vi "final16.vi"() -> ()   [LabVIEW 2019]
uses:
  <vilib>/Instr/_visa.llb/VISA Configure Serial Port (Instr).vi
  <vilib>/Analysis/NI_AALBase.lvlib
  <vilib>/Analysis/NI_AALPro.lvlib
panel:
  out "Noise":dbl
  out "Relative errors array":dbl[](array[numeric])
  out "Absolute errors array":dbl[](array[numeric])
  out "Calibration - read data":dbl[][](array[numeric])
  out "Received data":string[][](array[string])
  out "slope_gain0":dbl
  out "intercept_gain0":dbl
  out "residue_gain0":dbl
  out "slope_gain2":dbl
  out "intercept_gain2":dbl
  out "residue_gain2":dbl
  out "slope_gain1":dbl
  out "intercept_gain1":dbl
  out "residue_gain1":dbl
  out "standard deviation":dbl format="%0.2f"
  out "variance":dbl format="%0.2f"
  out "mean":dbl format="%0.2f"
  out "Conversion [g]":dbl
  out "String passed to Arduino":string
  out "Received data array":dbl[](array[numeric])
  out "Debug array":string[](array[string])
  in  "Stop":bool
  in  "Cycles":dbl min=1.0 step=1.0
  in  "Start operation":bool
  in  "Function":u16(ring) items=["Read data ", "Compare different gains", "Execute calibration"]
  in  "Gain":u16(ring) items=["32", "64", "128"]
  in  "Arduino COM port":refnum<visa-resource-name>="COM6"
  # "Select all options, then press \"Start operation\" button"
  # "Nerd zone"
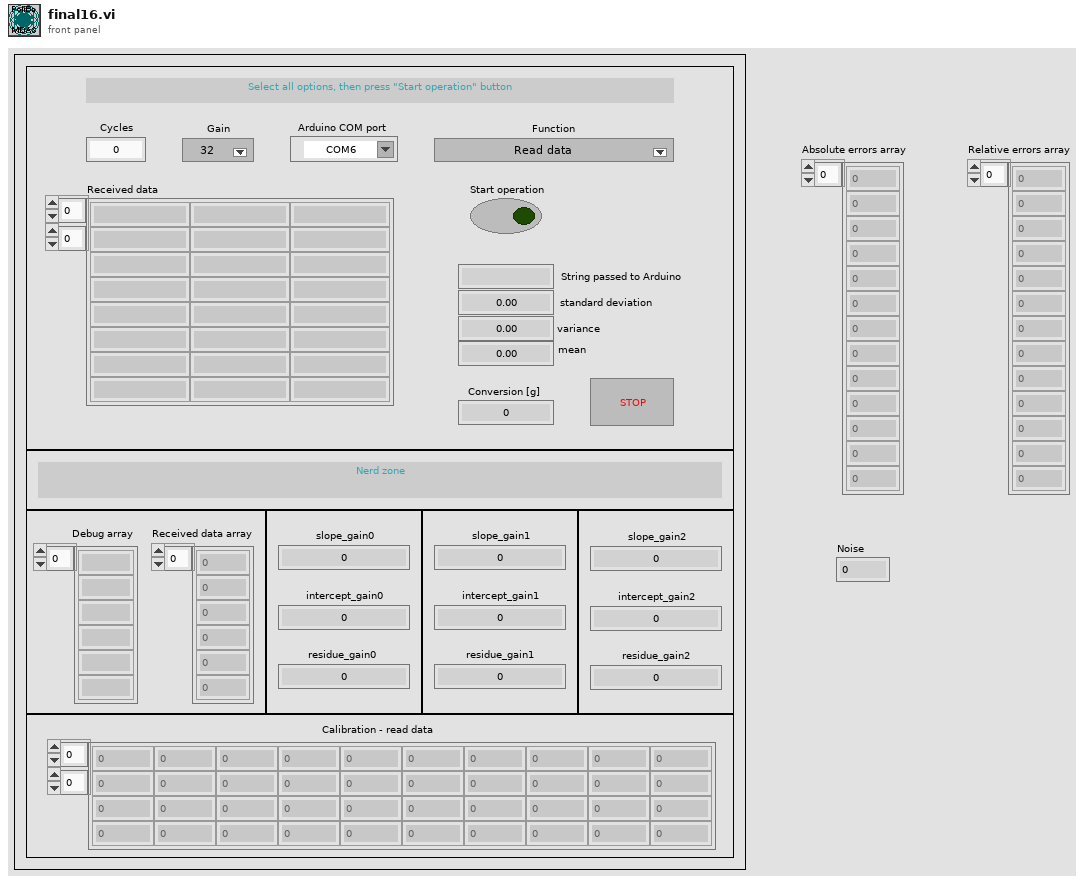
[diagram p1: front panel]
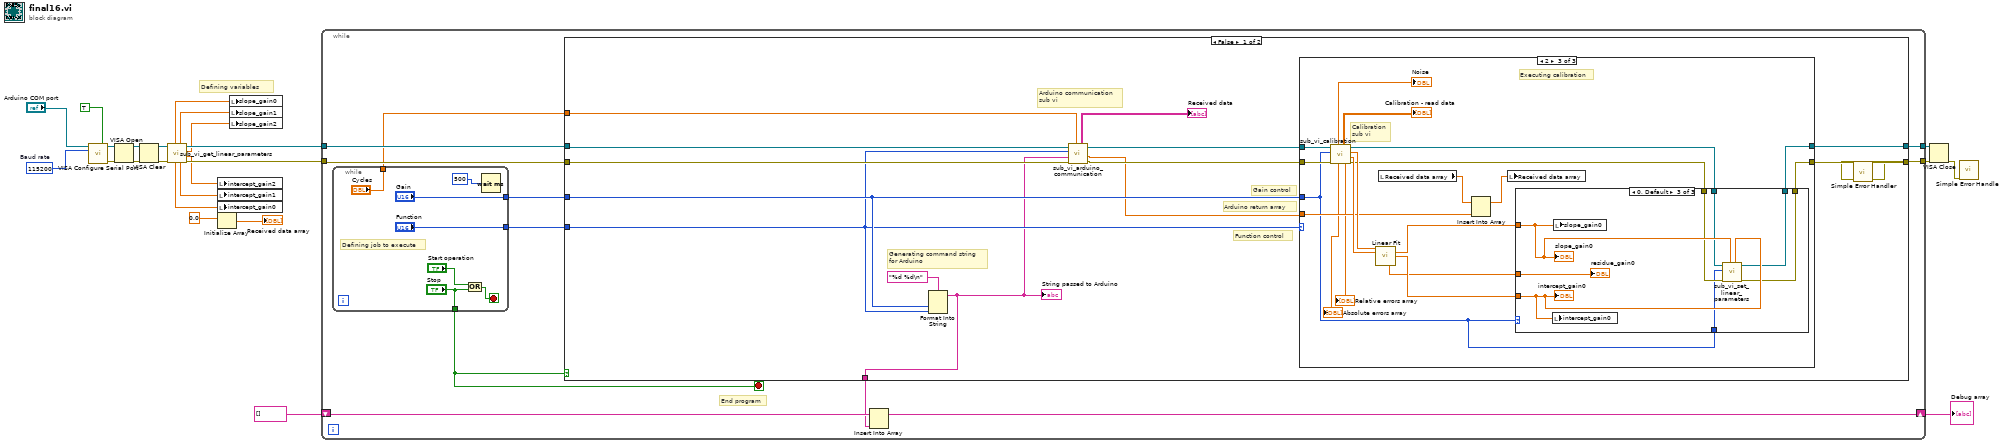
[diagram p0: block diagram]
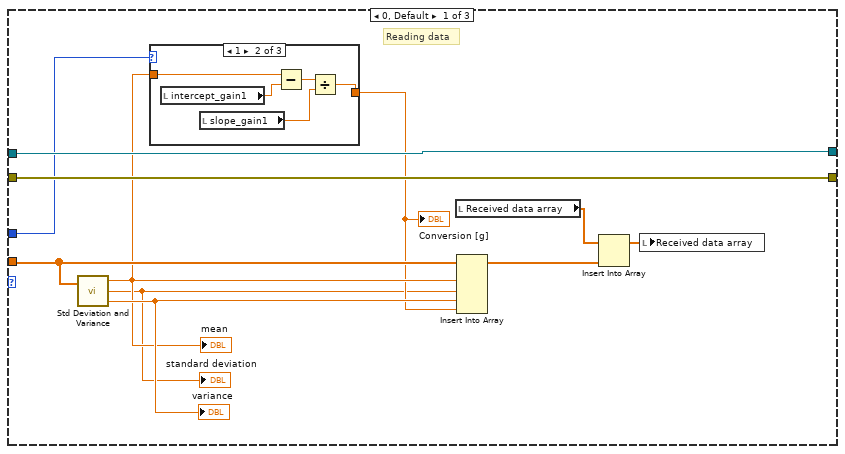
[diagram p2: hidden frame]
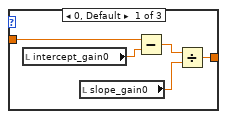
[diagram p3: hidden frame]
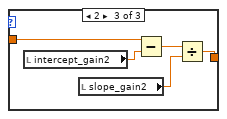
[diagram p4: hidden frame]
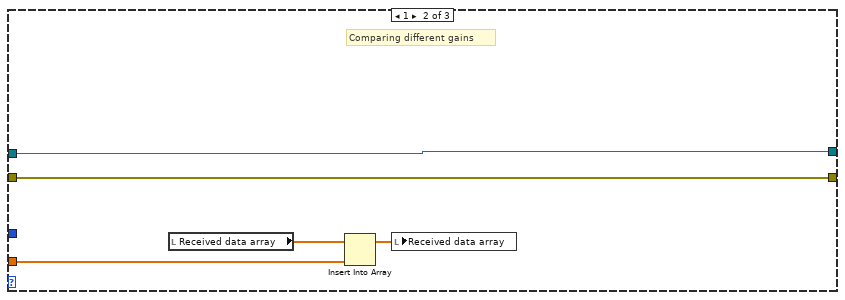
[diagram p5: hidden frame]
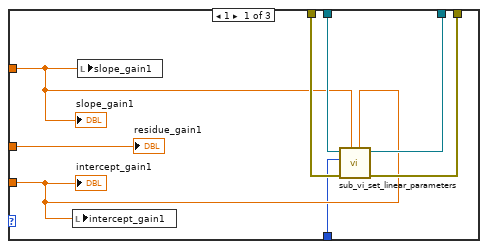
[diagram p6: hidden frame]
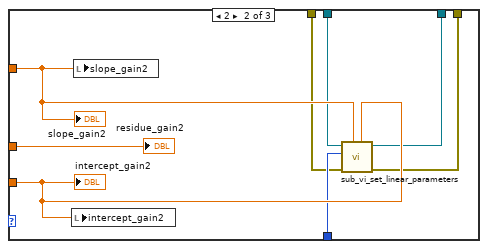
[diagram p7: hidden frame]
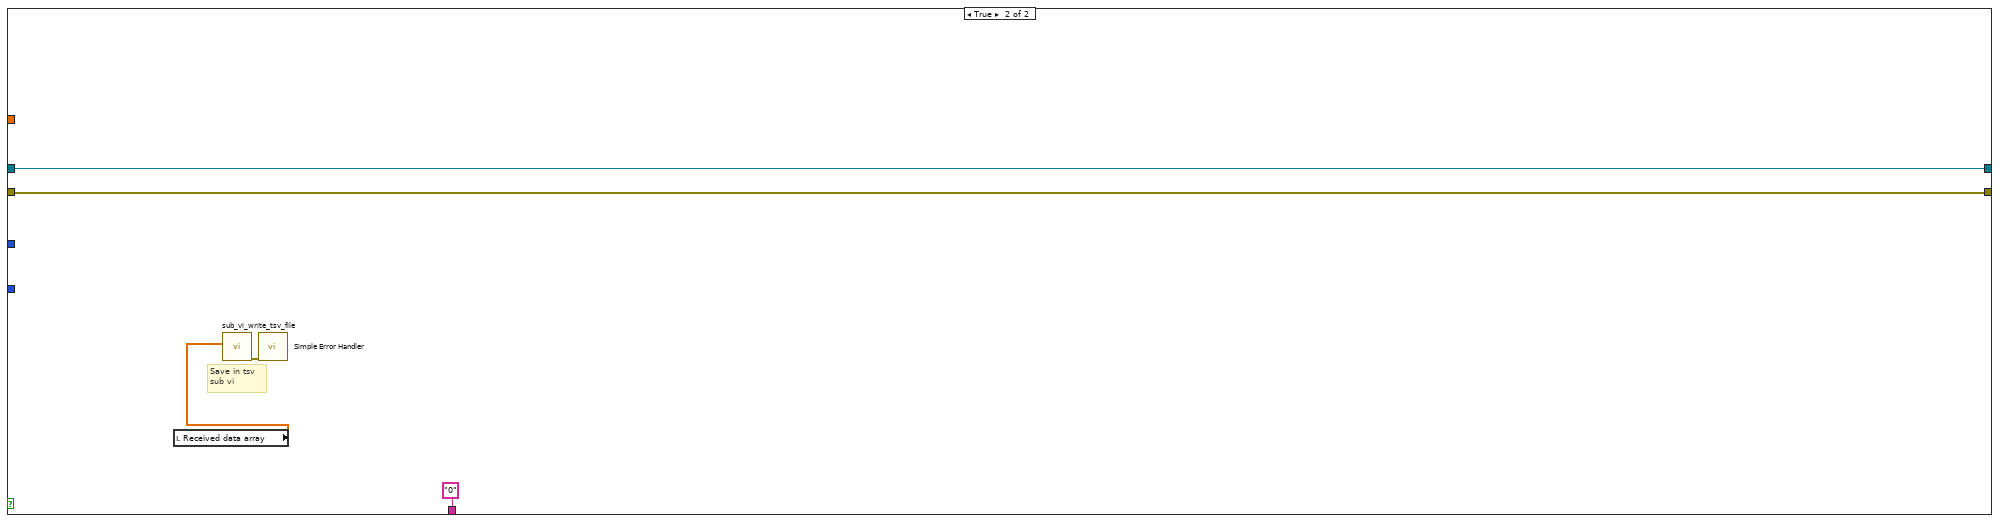
[diagram p8: hidden frame]
diagram:
  w23 = u32 115200  # Baud rate
  # "Defining variables"
  n1 = call-poly "VISA Configure Serial Port"("VISA resource name"="Arduino COM port", "Enable Termination\nChar (T)"=TRUE ("Enable Termination\nChar (T)"), "baud rate (9600)"=w23) -> ("VISA resource name out"=w21:refnum<visa-resource-name>, "error out"=w22:errorcluster)  [unwired: 11 in]
  n2 = VISA Open(error in (no error)=w22, VISA resource name=w21) -> (VISA resource name=w18:refnum<visa-resource-name>, error out=w19:errorcluster)  [unwired: 3 in]
  n3 = VISA Clear(VISA resource name=w18, error in (no error)=w19) -> (VISA resource name out=w6:refnum<visa-resource-name>, error out=w4:errorcluster)
  n4 = call "sub_vi_get_linear_parameters.vi"("error in"=w4, "VISA resource name in"=w6) -> ("error out"=w3:errorcluster, "intercept_2"=w2:dbl, "slope_2"=w1:dbl, "VISA resource name out"=w5:refnum<visa-resource-name>, "intercept_1"=w8:dbl, "slope_1"=w9:dbl, "intercept_0"=w7:dbl, "slope_0"=w10:dbl)  [unwired: 2 in]
  n5 = local write "intercept_gain2"(w2) -> ()
  n6 = local write "intercept_gain1"(w8) -> ()
  n7 = local write "intercept_gain0"(w7) -> ()
  n8 = Initialize Array(0.0) -> (→"Received data array":dbl[])  [unwired: 1 in]
  n9 = local write "slope_gain0"(w10) -> ()
  n10 = local write "slope_gain1"(w9) -> ()
  n11 = local write "slope_gain2"(w1) -> ()
  n12 = while {
    tunnel: w3 -> [w29]
    tunnel: w5 -> [w30]
    shift-right: [w35] -> w16
    shift-left: string[] [] -> [w33]
    tunnel: [w32] -> w12
    tunnel: [w31] -> w11
    stop <- w34 stop-if-true
    # "End program"
    n13 = while {
      tunnel: ["Function"] -> w26
      tunnel: ["Gain"] -> w27
      tunnel: ["Cycles"] -> w25
      tunnel: ["Stop"] -> w34
      stop <- w130 stop-if-true
      # "Defining job to execute"
      n14 = Or(x="Start operation", y="Stop") -> (x .or. y?=w130:bool)
      n15 = Wait (ms)(milliseconds to wait=u32 500) -> ()  [unwired: 1 out]
    }
    n16 = case shown="False" w34 {
      tunnel: [w36 w125] -> w32
      tunnel: [w48 w126] -> w31
      tunnel: w30 -> [w46 w126]
      tunnel: w29 -> [w45 w125]
      tunnel: [w39 "0"] -> w28
      tunnel: w27 -> [w47 _]
      tunnel: w26 -> [w40 _]
      tunnel: w25 -> [w38 _]
      frame False {
        # "Generating command string\nfor Arduino"
        # "Function control"
        # "Arduino return array"
        # "Gain control"
        # "Arduino communication\nsub vi"
        n17 = Format Into String(format string="%d %d\n", w47, w40) -> (resulting string=w39:string)  [unwired: 2 in, 1 out]
        "String passed to Arduino" <- w39
        n18 = call "sub_vi_arduino_communication.vi"("Cycles"=w38, "error in (no error)"=w45, "write buffer"=w39, "Function"=w40, "VISA resource name in"=w46) -> ("error out"=w44:errorcluster, "Reads array"=w42:dbl[], "VISA resource name out"=w43:refnum<visa-resource-name>, "Received data"=→"Received data":string[][])  [unwired: 1 in]
        n19 = case shown="2" w40 {
          tunnel: w47 -> [w52 _ w81]
          tunnel: w42 -> [w60 w78 w90]
          tunnel: w43 -> [w55 w80 w96]
          tunnel: w44 -> [w54 w79 w95]
          tunnel: [w55 w80 w84] -> w48
          tunnel: [w54 w79 w82] -> w37
          frame 0, Default {
            # "Reading data"
            n20 = call <vilib>:"Std Deviation and Variance.vi"("X"=w60) -> ("mean"=w53:dbl, "standard deviation"=w50:dbl, "variance"=w59:dbl)  [unwired: 1 in]
            "standard deviation" <- w50
            "variance" <- w59
            "mean" <- w53
            n21 = case shown="1" w52 {
              tunnel: [w64 w69 w74] -> w51
              tunnel: w53 -> [w61 w66 w71]
              frame 0, Default {
                n22 = local read "intercept_gain0"() -> (w63:dbl)
                n23 = local read "slope_gain0"() -> (w62:dbl)
                n24 = Subtract(x=w61, y=w63) -> (x-y=w65:dbl)
                n25 = Divide(x=w65, y=w62) -> (x/y=w64:dbl)
              }
              frame 1 {
                n26 = local read "intercept_gain1"() -> (w68:dbl)
                n27 = local read "slope_gain1"() -> (w67:dbl)
                n28 = Subtract(x=w66, y=w68) -> (x-y=w70:dbl)
                n29 = Divide(x=w70, y=w67) -> (x/y=w69:dbl)
              }
              frame 2 {
                n30 = local read "intercept_gain2"() -> (w73:dbl)
                n31 = local read "slope_gain2"() -> (w72:dbl)
                n32 = Subtract(x=w71, y=w73) -> (x-y=w75:dbl)
                n33 = Divide(x=w75, y=w72) -> (x/y=w74:dbl)
              }
            }
            "Conversion [g]" <- w51
            n34 = local read "Received data array"() -> (w57:dbl[])
            n35 = Insert Into Array(array=w60, new element #1=w53, new element #2=w50, new element #3=w59, new element #4=w51) -> (w56:dbl[])  [unwired: 1 in]
            n36 = Insert Into Array(array=w57, new element=w56) -> (w58:dbl[])  [unwired: 1 in]
            n37 = local write "Received data array"(w58) -> ()
          }
          frame 1 {
            # "Comparing different gains"
            n38 = local read "Received data array"() -> (w77:dbl[])
            n39 = Insert Into Array(array=w77, new element=w78) -> (w76:dbl[])  [unwired: 1 in]
            n40 = local write "Received data array"(w76) -> ()
          }
          frame 2 {
            # "Calibration\nsub vi"
            # "Executing calibration"
            n41 = call "sub_vi_calibration.vi"("error in (no error)"=w95, "Gain"=w81, "VISA resource name"=w96) -> ("error out"=w83:errorcluster, "Weights"=w94:dbl[], "Measures"=w93:dbl[], "VISA resource name out"=w85:refnum<visa-resource-name>, "Relative errors array"=→"Relative errors array":dbl[], "Calibration - read data"=→"Calibration - read data":dbl[][], "Absolute errors array"=→"Absolute errors array":dbl[], "Noise"=→"Noise":dbl)  [unwired: 1 in]
            n42 = call <vilib>:"Linear Fit.vi"("Y"=w93, "X"=w94) -> ("slope"=w99:dbl, "intercept"=w98:dbl, "residue"=w97:dbl)  [unwired: 9 in, 2 out]
            n43 = local read "Received data array"() -> (w91:dbl[])
            n44 = Insert Into Array(array=w91, new element=w90) -> (w92:dbl[])  [unwired: 1 in]
            n45 = local write "Received data array"(w92) -> ()
            n46 = case shown="0, Default" w81 {
              tunnel: w99 -> [w102 w114 w122]
              tunnel: w98 -> [w101 w113 w121]
              tunnel: w97 -> [w107 w115 w123]
              tunnel: w85 -> [w106 w111 w119]
              tunnel: [w104 w109 w120] -> w84
              tunnel: w83 -> [w105 w110 w118]
              tunnel: [w103 w108 w117] -> w82
              tunnel: w81 -> [w100 w112 w116]
              frame 1 {
                n47 = local write "intercept_gain1"(w101) -> ()
                n48 = local write "slope_gain1"(w102) -> ()
                n49 = call "sub_vi_set_linear_parameters.vi"("intercept"=w101, "slope"=w102, "error in (no error)"=w105, "gain"=w100, "VISA resource name in"=w106) -> ("error out"=w103:errorcluster, "VISA resource name out"=w104:refnum<visa-resource-name>)  [unwired: 5 in]
                "slope_gain1" <- w102
                "intercept_gain1" <- w101
                "residue_gain1" <- w107
              }
              frame 2 {
                n50 = local write "intercept_gain2"(w113) -> ()
                n51 = local write "slope_gain2"(w114) -> ()
                n52 = call "sub_vi_set_linear_parameters.vi"("intercept"=w113, "slope"=w114, "error in (no error)"=w110, "gain"=w112, "VISA resource name in"=w111) -> ("error out"=w108:errorcluster, "VISA resource name out"=w109:refnum<visa-resource-name>)  [unwired: 5 in]
                "slope_gain2" <- w114
                "intercept_gain2" <- w113
                "residue_gain2" <- w115
              }
              frame 0, Default {
                n53 = local write "intercept_gain0"(w121) -> ()
                n54 = local write "slope_gain0"(w122) -> ()
                n55 = call "sub_vi_set_linear_parameters.vi"("intercept"=w121, "slope"=w122, "error in (no error)"=w118, "gain"=w116, "VISA resource name in"=w119) -> ("error out"=w117:errorcluster, "VISA resource name out"=w120:refnum<visa-resource-name>)  [unwired: 5 in]
                "slope_gain0" <- w122
                "intercept_gain0" <- w121
                "residue_gain0" <- w123
              }
            }
          }
        }
        n56 = call <vilib>:"Simple Error Handler.vi"("error in (no error)"=w37) -> ("error out"=w36:errorcluster)  [unwired: 4 in, 4 out]
      }
      frame True {
        # "Save in tsv\nsub vi"
        n57 = local read "Received data array"() -> (w127:dbl[])
        n58 = call "sub_vi_write_tsv_file.vi"("1D data"=w127) -> ("error out"=w128:errorcluster)  [unwired: 10 in]
        n59 = call <vilib>:"Simple Error Handler.vi"("error in (no error)"=w128) -> ()  [unwired: 4 in, 5 out]
      }
    }
    n60 = Insert Into Array(array=w33, new element=w28) -> (w35:string[])  [unwired: 1 in]
  }
  "Debug array" <- w16
  n61 = VISA Close(VISA resource name=w11, error in (no error)=w12) -> (error out=w15:errorcluster)
  n62 = call <vilib>:"Simple Error Handler.vi"("error in (no error)"=w15) -> ()  [unwired: 4 in, 5 out]
